vi "PUERTOS DIG.vi"(0 "VISA resource name":refnum<visa-resource-name>, 5 "PUERTO":u8(ring) items=["PUERTOA", "PUERTOB", "PUERTOC", "PUERTOD", "PUERTOE"], 7 "OPERACION":u8(ring) items=["SALIDA", "ENTRADA"], 9 "DATO":u8, 11 "error":errorcluster, 12 "HABILITA":bool) -> (4 "VISA resource name":refnum<visa-resource-name>, 6 "RESULTADO":string, 8 "Resultado U8":u8, 15 "error":errorcluster)   [LabVIEW 2009]
panel:
  out "return count":u32
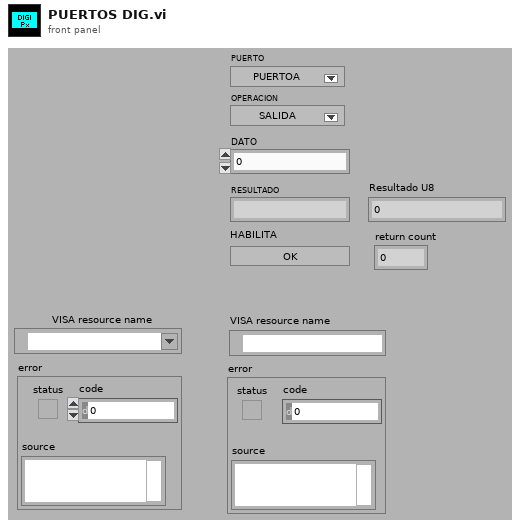
[diagram p1: front panel]
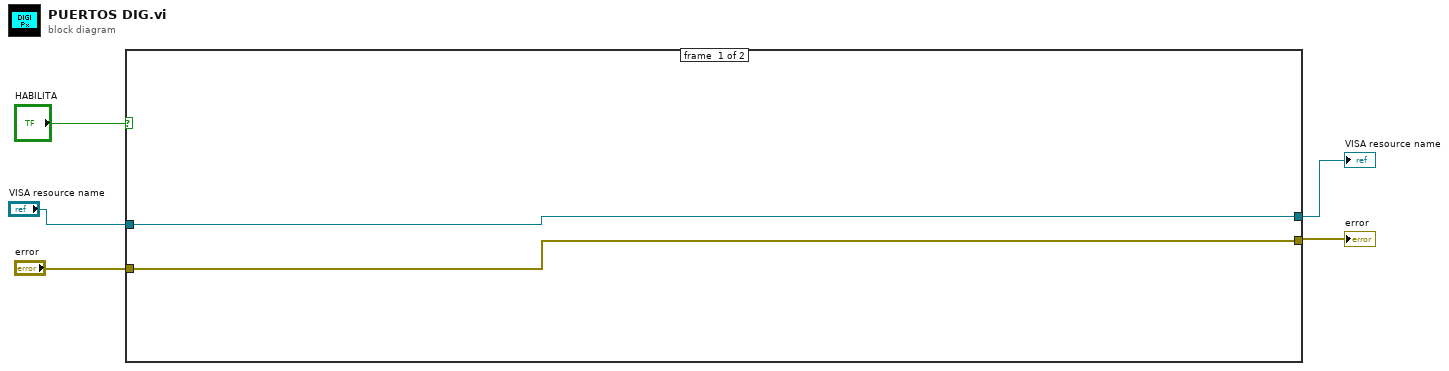
[diagram p0: block diagram]
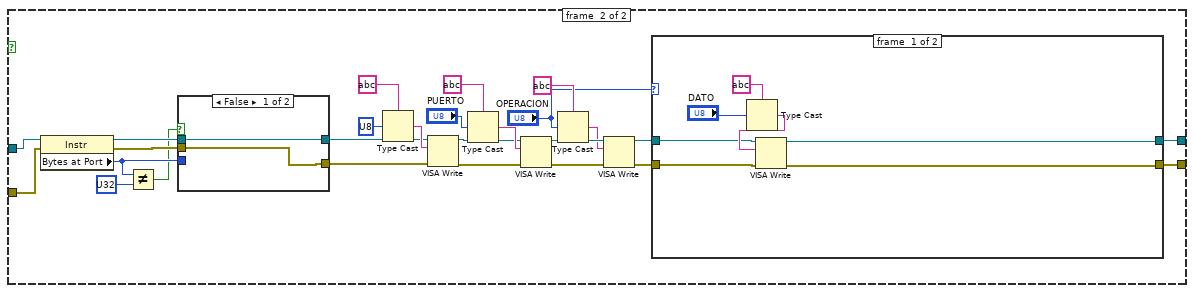
[diagram p2: hidden frame]
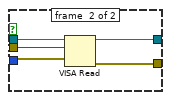
[diagram p3: hidden frame]
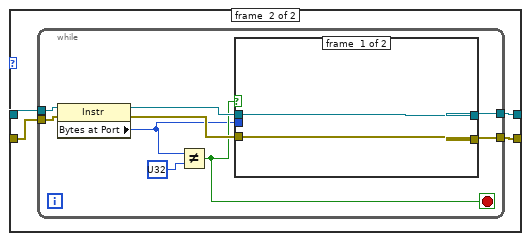
[diagram p4: hidden frame]
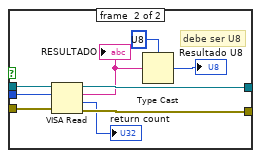
[diagram p5: hidden frame]
diagram:
  n1 = case shown="True" "HABILITA" {
    tunnel: "VISA resource name" -> [w7 w11]
    tunnel: "error" -> [w6 w12]
    tunnel: [w7 w33] -> w3
    tunnel: [w6 w32] -> w2
    frame #0 {
    }
    frame #1 {
      n2 = property class="Instr"(reference=w11, error in=w12) -> (reference out=w16:refnum<visa-resource-name>, error out=w15:errorcluster, "Bytes at Port"=w10:u32)
      n3 = Not Equal?(x=w10, y=u32 ?) -> (x != y?=w8:bool)
      n4 = case shown="False" w8 {
        tunnel: w16 -> [w35 w40]
        tunnel: w15 -> [w34 w39]
        tunnel: w10 -> [_ w38]
        tunnel: [w35 w37] -> w14
        tunnel: [w34 w36] -> w13
        frame #0 {
        }
        frame #1 {
          n5 = VISA Read(VISA resource name=w40, byte count=w38, error in (no error)=w39) -> (VISA resource name out=w37:refnum<visa-resource-name>, error out=w36:errorcluster)  [unwired: 2 out]
        }
      }
      n6 = Type Cast(type=string ?, x=u8 ?) -> (*(type *) &x=w20:string)
      n7 = VISA Write(VISA resource name=w14, write buffer=w20, error in (no error)=w13) -> (VISA resource name out=w21:refnum<visa-resource-name>, error out=w22:errorcluster)  [unwired: 1 out]
      n8 = Type Cast(type=string ?, x="PUERTO") -> (*(type *) &x=w26:string)
      n9 = VISA Write(VISA resource name=w21, write buffer=w26, error in (no error)=w22) -> (VISA resource name out=w31:refnum<visa-resource-name>, error out=w30:errorcluster)  [unwired: 1 out]
      n10 = Type Cast(type=string ?, x="OPERACION") -> (*(type *) &x=w28:string)
      n11 = VISA Write(VISA resource name=w31, write buffer=w28, error in (no error)=w30) -> (VISA resource name out=w19:refnum<visa-resource-name>, error out=w18:errorcluster)  [unwired: 1 out]
      n12 = case shown="1" "OPERACION" {
        tunnel: [w42 w51] -> w33
        tunnel: [w41 w50] -> w32
        tunnel: w19 -> [w44 w49]
        tunnel: w18 -> [w43 w48]
        frame #0 {
          n13 = Type Cast(type=string ?, x="DATO") -> (*(type *) &x=w46:string)
          n14 = VISA Write(VISA resource name=w44, write buffer=w46, error in (no error)=w43) -> (VISA resource name out=w42:refnum<visa-resource-name>, error out=w41:errorcluster)  [unwired: 1 out]
        }
        frame #1 {
          n15 = while {
            tunnel: [w60] -> w51
            tunnel: [w59] -> w50
            tunnel: w49 -> [w56]
            tunnel: w48 -> [w55]
            stop <- w53 stop-if-true
            n16 = property class="Instr"(reference=w56, error in=w55) -> (reference out=w58:refnum<visa-resource-name>, error out=w57:errorcluster, "Bytes at Port"=w52:u32)
            n17 = Not Equal?(x=w52, y=u32 ?) -> (x != y?=w53:bool)
            n18 = case shown="True" w53 {
              tunnel: [w62 w71] -> w60
              tunnel: [w61 w70] -> w59
              tunnel: w58 -> [w62 w69]
              tunnel: w57 -> [w61 w68]
              tunnel: w52 -> [_ w63]
              frame #0 {
              }
              frame #1 {
                # "debe ser U8"
                n19 = VISA Read(VISA resource name=w69, byte count=w63, error in (no error)=w68) -> (VISA resource name out=w71:refnum<visa-resource-name>, read buffer=w67:string, return count=→"return count":u32, error out=w70:errorcluster)
                "RESULTADO" <- w67
                n20 = Type Cast(type=u8 ?, x=w67) -> (*(type *) &x=→"Resultado U8":u8)
              }
            }
          }
        }
      }
    }
  }
  "VISA resource name" <- w3
  "error" <- w2
